vi "TheGameUserInterface.vi"() -> ()   [LabVIEW 2014]
uses:
  <vilib>/addons/Multicore Analysis and Sparse Matrix/Statistics/_statistics/Mean (DBL).vi
  <vilib>/addons/Multicore Analysis and Sparse Matrix/Statistics/NI_MASM_Statistics.lvlib
panel:
  out "a":dbl[][](array[numeric])
  in  "Boolean":bool
  out "String":string
  in  "stop":bool
  in  "Enum":enum16{"Calibrate", "Play"}(ring)
  out "Draw?":bool
  out "Player 1 win":bool
  out "Player 2 win":bool
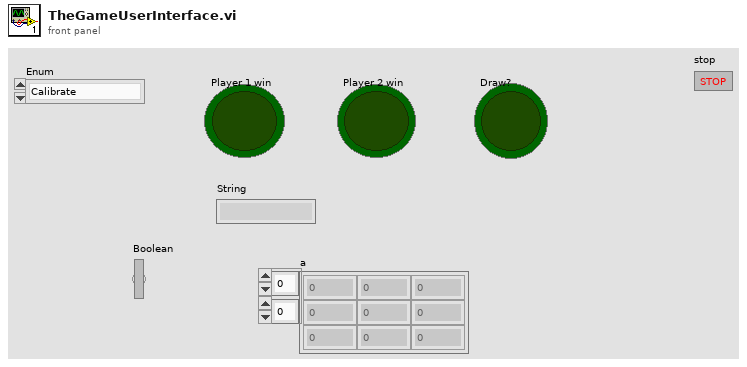
[diagram p1: front panel]
types:
  T1 = enum16{"open", "replace", "create", "open or create", "replace or create", "replace or create with confirmation"}
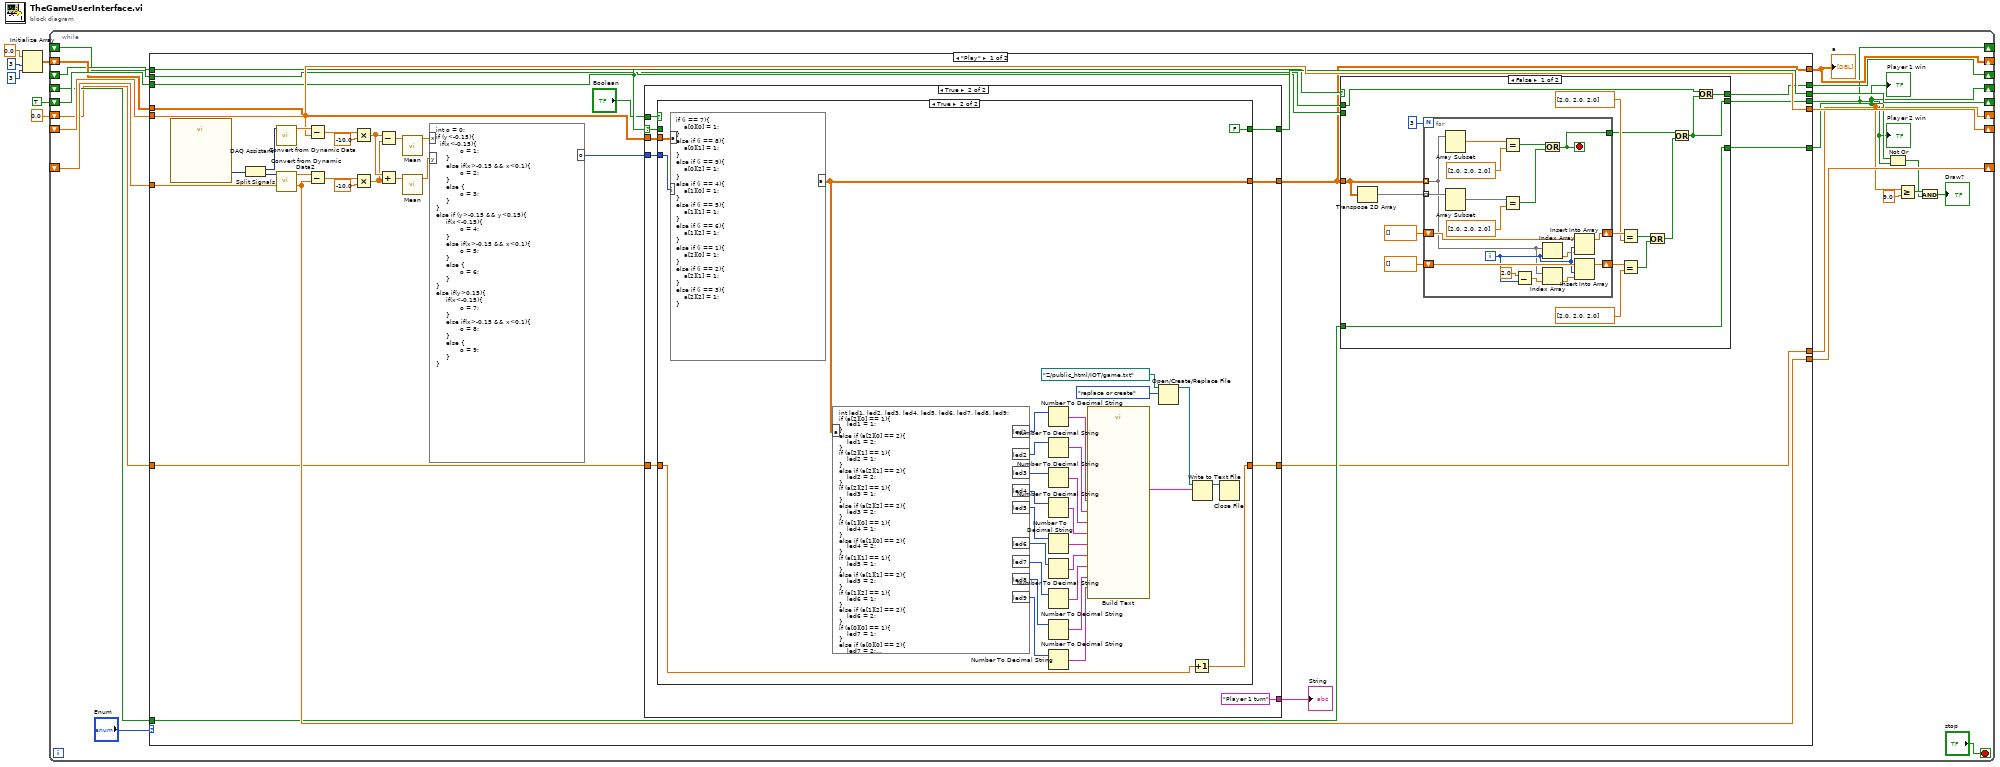
[diagram p0: block diagram]
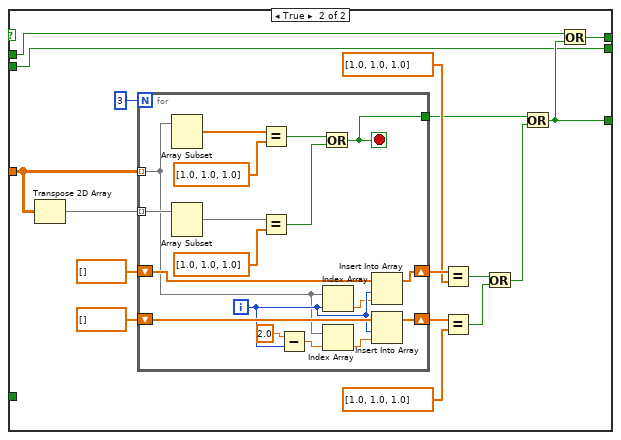
[diagram p2: hidden frame]
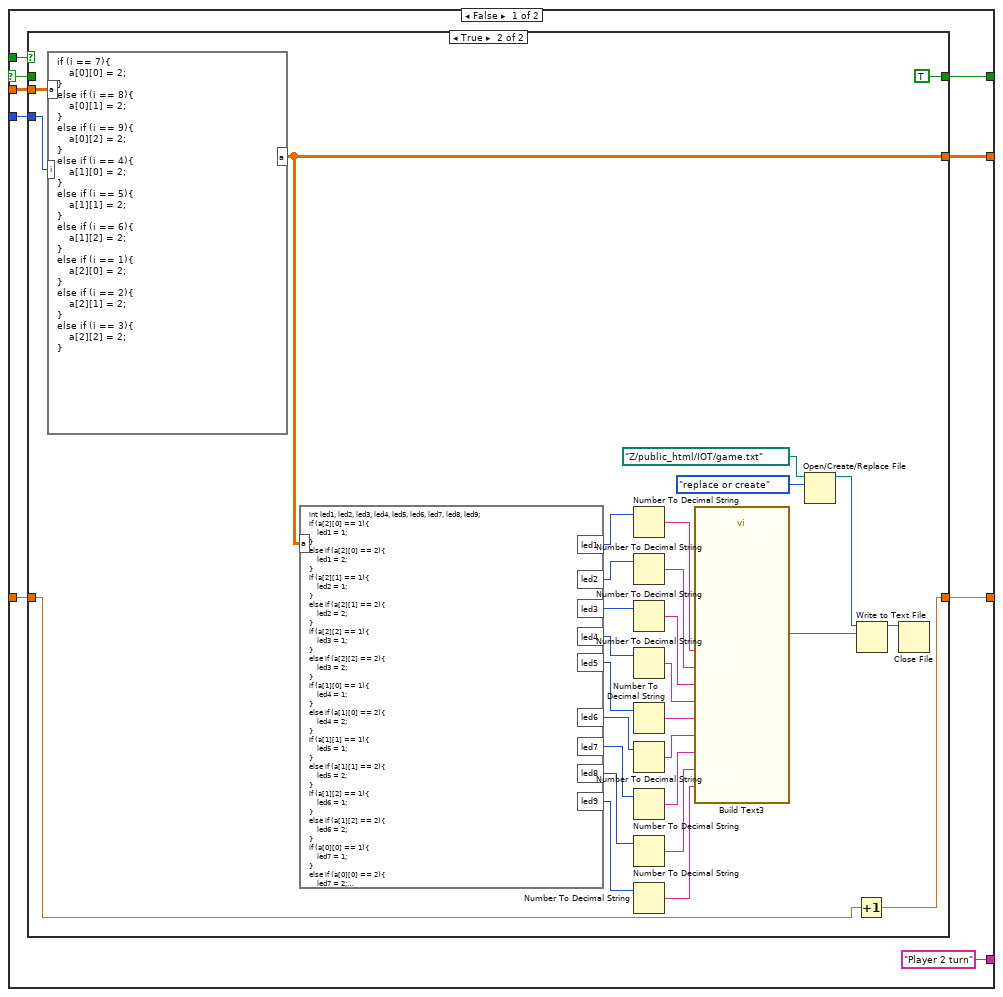
[diagram p3: hidden frame]
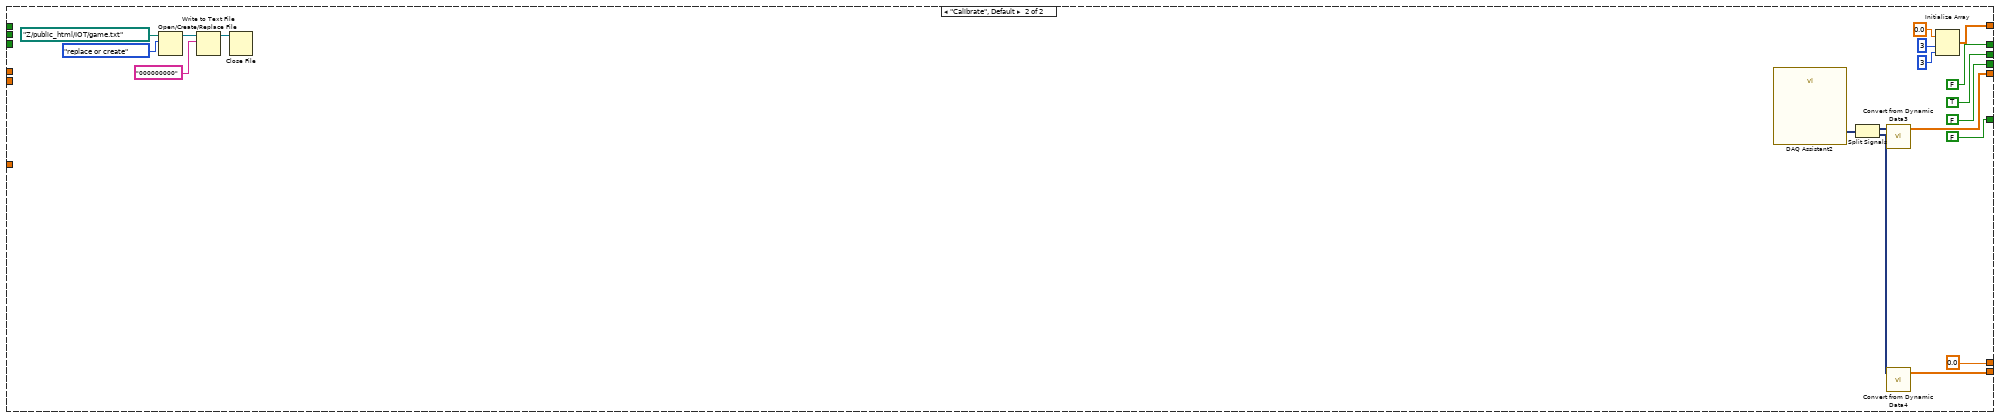
[diagram p6: hidden frame]
diagram:
  n1 = Initialize Array(0.0 ("element"), 3 ("dimension size"), 3 ("dimension size")) -> (w3:dbl[][])
  n2 = while {
    shift-right: [w24] -> _
    shift-left: _ -> [w28]
    shift-right: [w23] -> _
    shift-left: _ -> [w27]
    shift-right: [w22] -> _
    shift-left: w3 -> [w19]
    shift-right: [w20] -> _
    shift-left: TRUE -> [w21]
    shift-right: [w18] -> _
    shift-left: _ -> [w17]
    shift-right: [w14] -> _
    shift-left: _ -> [w16]
    shift-right: [w13] -> _
    shift-left: _ -> [w15]
    shift-right: [w11] -> _
    shift-left: 0.0 ("element") -> [w12]
    stop <- "stop" stop-if-true
    n3 = case shown="\"Play\"" "Enum" {
      tunnel: [w46 w229] -> w24
      tunnel: [w45 w228] -> w23
      tunnel: w28 -> [w46 _]
      tunnel: w27 -> [w45 _]
      tunnel: w19 -> [w41 _]
      tunnel: [w30 w223] -> w22
      tunnel: w21 -> [w42 _]
      tunnel: [w43 TRUE] -> w20
      tunnel: [w40 FALSE] -> w18
      tunnel: w17 -> [w39 _]
      tunnel: [w38 FALSE] -> w14
      tunnel: [w37 FALSE] -> w13
      tunnel: w16 -> [w36 _]
      tunnel: w15 -> [w35 _]
      tunnel: w12 -> [w34 _]
      tunnel: [w33 0.0 ("element")] -> w11
      frame "Play" {
        n4 = call "DAQ Assistant"() -> ("data"=w31:dynamicdata)  [unwired: 17 in, 2 out]
        n5 = Split Signals(w31) -> (w56:dynamicdata, w55:dynamicdata)  [unwired: 2 in]
        n6 = call "Convert from Dynamic Data"("Dynamic Data Type"=w56) -> ("Array"=w48:dbl[])  [unwired: 3 in]
        n7 = call "Convert from Dynamic Data2"("Dynamic Data Type"=w55) -> ("Array"=w47:dbl[])  [unwired: 3 in]
        n8 = Subtract(x=w48, y=w46) -> (x-y=w50:dbl[])
        n9 = Subtract(x=w47, y=w45) -> (x-y=w49:dbl[])
        n10 = Multiply(x=w50, y=-10.0) -> (x*y=w58:dbl[])
        n11 = Multiply(x=w49, y=-10.0) -> (x*y=w57:dbl[])
        n12 = Subtract(x=w58, y=w57) -> (x-y=w54:dbl[])
        n13 = Add(x=w58, y=w57) -> (x+y=w53:dbl[])
        n14 = call-poly <vilib>:"Mean.vi"("X"=w54) -> ("mean"=w52:dbl)  [unwired: 9 in, 1 out]
        n15 = call-poly <vilib>:"Mean.vi"("X"=w53) -> ("mean"=w51:dbl)  [unwired: 9 in, 1 out]
        n16 = formula code="int o = 0;\nif (y<-0.15){\n  if(x<-0.15){\n            o = 1;\n     }\n     else if(x>-0.15 && x<0.1){\n            o = 2;\n     }\n     else {\n            o = 3;\n     }\n}\nelse if (y>-0.15 && y<0.15){\n     if(x<-0.15){\n            o = 4;\n     }\n     else if(x>-0.15 && x<0.1){\n            o = 5;\n     }\n     else {\n            o = 6;\n     }\n}\nelse if(y>0.15){\n     if(x<-0.15){\n            o = 7;\n     }\n     else if(x>-0.15 && x<0.1){\n            o = 8;\n     }\n     else {\n            o = 9;\n     }\n}"("x"=w52, "y"=w51) -> ("o"=w44:i32)
        n17 = case shown="True" w42 {
          selector: w42 -> [w132 w173]
          tunnel: w44 -> [w138 w180]
          tunnel: w41 -> [w139 w179]
          tunnel: [w136 w178] -> w30
          tunnel: "Boolean" -> [w137 w177]
          tunnel: [w135 w176] -> w43
          tunnel: w34 -> [w134 w175]
          tunnel: [w133 w174] -> w33
          tunnel: ["Player 2 turn" ("String") "Player 1 turn" ("String")] -> w32
          frame False {
            n18 = case shown="True" w137 {
              tunnel: [w142 w143] -> w136
              tunnel: w139 -> [w142 w171]
              tunnel: w138 -> [_ w170]
              tunnel: [w141 TRUE] -> w135
              tunnel: w132 -> [w141 _]
              tunnel: w134 -> [w140 w168]
              tunnel: [w140 w167] -> w133
              frame False {
              }
              frame True {
                n19 = formula code="if (i == 7){\n    a[0][0] = 2;\n}\nelse if (i == 8){\n    a[0][1] = 2;\n}\nelse if (i == 9){\n    a[0][2] = 2;\n}\nelse if (i == 4){\n    a[1][0] = 2;\n}\nelse if (i == 5){\n    a[1][1] = 2;\n}\nelse if (i == 6){\n    a[1][2] = 2;\n}\nelse if (i == 1){\n    a[2][0] = 2;\n}\nelse if (i == 2){\n    a[2][1] = 2;\n}\nelse if (i == 3){\n    a[2][2] = 2;\n}"("i"=w170, "a"=w171) -> ("a"=w143:dbl[][])
                n20 = formula code="int led1, led2, led3, led4, led5, led6, led7, led8, led9;\nif (a[2][0] == 1){\n    led1 = 1;\n}\nelse if (a[2][0] == 2){\n    led1 = 2;\n}\nif (a[2][1] == 1){\n    led2 = 1;\n}\nelse if (a[2][1] == 2){\n    led2 = 2;\n}\nif (a[2][2] == 1){\n    led3 = 1;\n}\nelse if (a[2][2] == 2){\n    led3 = 2;\n}\nif (a[1][0] == 1){\n    led4 = 1;\n}\nelse if (a[1][0] == 2){\n    led4 = 2;\n}\nif (a[1][1] == 1){\n    led5 = 1;\n}\nelse if (a[1][1] == 2){\n    led5 = 2;\n}\nif (a[1][2] == 1){\n    led6 = 1;\n}\nelse if (a[1][2] == 2){\n    led6 = 2;\n}\nif (a[0][0] == 1){\n    led7 = 1;\n}\nelse if (a[0][0] == 2){\n    led7 = 2;\n}\nif (a[0][1] == 1){\n    led8 = 1;\n}\nelse if (a[0][1] == 2){\n    led8 = 2;\n}\nif (a[0][2] == 1){\n    led9 = 1;\n}\nelse if (a[0][2] == 2){\n    led9 = 2;\n}"("a"=w143) -> ("led1"=w165:i32, "led2"=w163:i32, "led3"=w162:i32, "led4"=w161:i32, "led5"=w160:i32, "led6"=w159:i32, "led7"=w158:i32, "led8"=w157:i32, "led9"=w156:i32)
                n21 = Number To Decimal String(number=w165) -> (decimal integer string=w164:string)  [unwired: 1 in]
                n22 = Number To Decimal String(number=w163) -> (decimal integer string=w155:string)  [unwired: 1 in]
                n23 = Number To Decimal String(number=w162) -> (decimal integer string=w154:string)  [unwired: 1 in]
                n24 = Number To Decimal String(number=w161) -> (decimal integer string=w153:string)  [unwired: 1 in]
                n25 = Number To Decimal String(number=w160) -> (decimal integer string=w152:string)  [unwired: 1 in]
                n26 = Number To Decimal String(number=w159) -> (decimal integer string=w151:string)  [unwired: 1 in]
                n27 = Number To Decimal String(number=w158) -> (decimal integer string=w150:string)  [unwired: 1 in]
                n28 = Number To Decimal String(number=w157) -> (decimal integer string=w149:string)  [unwired: 1 in]
                n29 = Number To Decimal String(number=w156) -> (decimal integer string=w148:string)  [unwired: 1 in]
                n30 = call "Build Text3"("Led1"=w164, "Led2"=w155, "Led3"=w154, "Led4"=w153, "Led5"=w152, "Led6"=w151, "Led7"=w150, "Led8"=w149, "Led9"=w148) -> ("Result"=w166:string)  [unwired: 17 in, 1 out]
                n31 = Open/Create/Replace File(file path (use dialog)=path "Z:/public_html/IOT/game.txt", operation (0:open)=T1."replace or create") -> (refnum out=w145:refnum<file>)  [unwired: 4 in, 2 out]
                n32 = Increment(x=w168) -> (x+1=w167:dbl)
                n33 = Write to Text File(file (use dialog)=w145, text=w166) -> (refnum out=w144:refnum<file>)  [unwired: 2 in, 2 out]
                n34 = Close File(refnum=w144) -> ()  [unwired: 1 in, 2 out]
              }
            }
          }
          frame True {
            n35 = case shown="True" w177 {
              tunnel: w180 -> [_ w212]
              tunnel: [w183 w184] -> w178
              tunnel: w179 -> [w183 w211]
              tunnel: [w182 FALSE] -> w176
              tunnel: w173 -> [w182 _]
              tunnel: w175 -> [w181 w209]
              tunnel: [w181 w208] -> w174
              frame False {
              }
              frame True {
                n36 = formula code="if (i == 7){\n    a[0][0] = 1;\n}\nelse if (i == 8){\n    a[0][1] = 1;\n}\nelse if (i == 9){\n    a[0][2] = 1;\n}\nelse if (i == 4){\n    a[1][0] = 1;\n}\nelse if (i == 5){\n    a[1][1] = 1;\n}\nelse if (i == 6){\n    a[1][2] = 1;\n}\nelse if (i == 1){\n    a[2][0] = 1;\n}\nelse if (i == 2){\n    a[2][1] = 1;\n}\nelse if (i == 3){\n    a[2][2] = 1;\n}"("i"=w212, "a"=w211) -> ("a"=w184:dbl[][])
                n37 = formula code="int led1, led2, led3, led4, led5, led6, led7, led8, led9;\nif (a[2][0] == 1){\n    led1 = 1;\n}\nelse if (a[2][0] == 2){\n    led1 = 2;\n}\nif (a[2][1] == 1){\n    led2 = 1;\n}\nelse if (a[2][1] == 2){\n    led2 = 2;\n}\nif (a[2][2] == 1){\n    led3 = 1;\n}\nelse if (a[2][2] == 2){\n    led3 = 2;\n}\nif (a[1][0] == 1){\n    led4 = 1;\n}\nelse if (a[1][0] == 2){\n    led4 = 2;\n}\nif (a[1][1] == 1){\n    led5 = 1;\n}\nelse if (a[1][1] == 2){\n    led5 = 2;\n}\nif (a[1][2] == 1){\n    led6 = 1;\n}\nelse if (a[1][2] == 2){\n    led6 = 2;\n}\nif (a[0][0] == 1){\n    led7 = 1;\n}\nelse if (a[0][0] == 2){\n    led7 = 2;\n}\nif (a[0][1] == 1){\n    led8 = 1;\n}\nelse if (a[0][1] == 2){\n    led8 = 2;\n}\nif (a[0][2] == 1){\n    led9 = 1;\n}\nelse if (a[0][2] == 2){\n    led9 = 2;\n}"("a"=w184) -> ("led1"=w206:i32, "led2"=w204:i32, "led3"=w203:i32, "led4"=w202:i32, "led5"=w201:i32, "led6"=w200:i32, "led7"=w199:i32, "led8"=w198:i32, "led9"=w197:i32)
                n38 = Number To Decimal String(number=w206) -> (decimal integer string=w205:string)  [unwired: 1 in]
                n39 = Number To Decimal String(number=w204) -> (decimal integer string=w196:string)  [unwired: 1 in]
                n40 = Number To Decimal String(number=w203) -> (decimal integer string=w195:string)  [unwired: 1 in]
                n41 = Number To Decimal String(number=w202) -> (decimal integer string=w194:string)  [unwired: 1 in]
                n42 = Number To Decimal String(number=w201) -> (decimal integer string=w193:string)  [unwired: 1 in]
                n43 = Number To Decimal String(number=w200) -> (decimal integer string=w192:string)  [unwired: 1 in]
                n44 = Number To Decimal String(number=w199) -> (decimal integer string=w191:string)  [unwired: 1 in]
                n45 = Number To Decimal String(number=w198) -> (decimal integer string=w190:string)  [unwired: 1 in]
                n46 = Number To Decimal String(number=w197) -> (decimal integer string=w189:string)  [unwired: 1 in]
                n47 = call "Build Text"("Led1"=w205, "Led2"=w196, "Led3"=w195, "Led4"=w194, "Led5"=w193, "Led6"=w192, "Led7"=w191, "Led8"=w190, "Led9"=w189) -> ("Result"=w207:string)  [unwired: 17 in, 1 out]
                n48 = Open/Create/Replace File(file path (use dialog)=path "Z:/public_html/IOT/game.txt", operation (0:open)=T1."replace or create") -> (refnum out=w186:refnum<file>)  [unwired: 4 in, 2 out]
                n49 = Increment(x=w209) -> (x+1=w208:dbl)
                n50 = Write to Text File(file (use dialog)=w186, text=w207) -> (refnum out=w185:refnum<file>)  [unwired: 2 in, 2 out]
                n51 = Close File(refnum=w185) -> ()  [unwired: 1 in, 2 out]
              }
            }
          }
        }
        "String" <- w32
        n52 = case shown="False" w42 {
          tunnel: w30 -> [w65 w100]
          tunnel: [w63 w98] -> w40
          tunnel: w39 -> [w64 w99]
          tunnel: [w61 w97] -> w38
          tunnel: [w62 w96] -> w37
          tunnel: w36 -> [w61 _]
          tunnel: w35 -> [_ w96]
          frame False {
            n53 = Transpose 2D Array(2D array=w65) -> (transposed array=w76:dbl[][])
            n54 = for {
              N: 3 ("Numeric") -> [_]
              tunnel: w76 -> [w82] mode=indexing
              shift-right: [w89] -> w74
              shift-left: dbl[] [] ("array 4") -> [w90]
              tunnel: [w88] -> w66
              shift-right: [w83] -> w70
              shift-left: dbl[] [] ("array 5") -> [w85]
              tunnel: w65 -> [w80] mode=indexing
              i -> [w84]
              stop <- w88 stop-if-true
              n55 = Array Subset(array=w80) -> (w78:dbl[])  [unwired: 2 in]
              n56 = Array Subset(array=w82) -> (w94:dbl[])  [unwired: 2 in]
              n57 = Equal?(x=w78, y=dbl[] [2.0, 2.0, 2.0]) -> (x = y?=w92:bool)
              n58 = Equal?(x=w94, y=dbl[] [2.0, 2.0, 2.0]) -> (x = y?=w91:bool)
              n59 = Subtract(x=2.0, y=w84) -> (x-y=w86:dbl)
              n60 = Or(x=w92, y=w91) -> (x .or. y?=w88:bool)
              n61 = Index Array(array=w80, index=w84) -> (element=w81:dbl)
              n62 = Index Array(array=w80, index=w86) -> (element=w79:dbl)
              n63 = Insert Into Array(array=w90, index=w84, new element=w81) -> (w89:dbl[])
              n64 = Insert Into Array(array=w85, index=w84, new element=w79) -> (w83:dbl[])
            }
            n65 = Equal?(x=w74, y=dbl[] [2.0, 2.0, 2.0]) -> (x = y?=w69:bool)
            n66 = Equal?(x=w70, y=dbl[] [2.0, 2.0, 2.0]) -> (x = y?=w68:bool)
            n67 = Or(x=w69, y=w68) -> (x .or. y?=w67:bool)
            n68 = Or(x=w66, y=w67) -> (x .or. y?=w62:bool)
            n69 = Or(x=w64, y=w62) -> (x .or. y?=w63:bool)
          }
          frame True {
            n70 = Transpose 2D Array(2D array=w100) -> (transposed array=w111:dbl[][])
            n71 = for {
              N: 3 ("Numeric") -> [_]
              tunnel: w111 -> [w117] mode=indexing
              shift-right: [w124] -> w109
              shift-left: dbl[] [] ("array") -> [w125]
              tunnel: [w123] -> w101
              shift-right: [w118] -> w105
              shift-left: dbl[] [] ("array 2") -> [w120]
              tunnel: w100 -> [w115] mode=indexing
              i -> [w119]
              stop <- w123 stop-if-true
              n72 = Array Subset(array=w115) -> (w113:dbl[])  [unwired: 2 in]
              n73 = Array Subset(array=w117) -> (w129:dbl[])  [unwired: 2 in]
              n74 = Equal?(x=w113, y=dbl[] [1.0, 1.0, 1.0]) -> (x = y?=w127:bool)
              n75 = Equal?(x=w129, y=dbl[] [1.0, 1.0, 1.0]) -> (x = y?=w126:bool)
              n76 = Subtract(x=2.0, y=w119) -> (x-y=w121:dbl)
              n77 = Or(x=w127, y=w126) -> (x .or. y?=w123:bool)
              n78 = Index Array(array=w115, index=w119) -> (element=w116:dbl)
              n79 = Index Array(array=w115, index=w121) -> (element=w114:dbl)
              n80 = Insert Into Array(array=w125, index=w119, new element=w116) -> (w124:dbl[])
              n81 = Insert Into Array(array=w120, index=w119, new element=w114) -> (w118:dbl[])
            }
            n82 = Equal?(x=w109, y=dbl[] [1.0, 1.0, 1.0]) -> (x = y?=w104:bool)
            n83 = Equal?(x=w105, y=dbl[] [1.0, 1.0, 1.0]) -> (x = y?=w103:bool)
            n84 = Or(x=w104, y=w103) -> (x .or. y?=w102:bool)
            n85 = Or(x=w101, y=w102) -> (x .or. y?=w97:bool)
            n86 = Or(x=w99, y=w97) -> (x .or. y?=w98:bool)
          }
        }
      }
      frame "Calibrate", Default {
        n87 = Open/Create/Replace File(file path (use dialog)=path "Z:/public_html/IOT/game.txt", operation (0:open)=T1."replace or create") -> (refnum out=w215:refnum<file>)  [unwired: 4 in, 2 out]
        n88 = Write to Text File(file (use dialog)=w215, text="000000000") -> (refnum out=w214:refnum<file>)  [unwired: 2 in, 2 out]
        n89 = Close File(refnum=w214) -> ()  [unwired: 1 in, 2 out]
        n90 = call "DAQ Assistant2"() -> ("data"=w218:dynamicdata)  [unwired: 17 in, 2 out]
        n91 = Split Signals(w218) -> (w231:dynamicdata, w230:dynamicdata)  [unwired: 2 in]
        n92 = call "Convert from Dynamic Data3"("Dynamic Data Type"=w231) -> ("Array"=w229:dbl[])  [unwired: 3 in]
        n93 = call "Convert from Dynamic Data4"("Dynamic Data Type"=w230) -> ("Array"=w228:dbl[])  [unwired: 3 in]
        n94 = Initialize Array(0.0 ("element"), 3 ("dimension size"), 3 ("dimension size")) -> (w223:dbl[][])
      }
    }
    "Player 1 win" <- w14
    "Player 2 win" <- w13
    "a" <- w22
    n95 = Not Or(1:w13, 2:w14) -> (0:w8:bool)
    n96 = Greater Or Equal?(x=w11, y=9.0) -> (x >= y?=w9:bool)
    n97 = And(x=w9, y=w8) -> (x .and. y?=→"Draw?":bool)
  }
